vi "RT_DETR_OpenVINO.vi"() -> ()   [LabVIEW 2018]
doc: "RT_DETR_OpenVINO: This example is an object detection example of the RT-DETR algorithm, which can perform object detection on real-time images captured by cameras."
uses:
  vi.lib/VIRobotics/opencv_yiku/Cap/Cap.lvclass
  vi.lib/VIRobotics/ModelZoo/Object_Detection/RT_DETR_OpenVINO/RT_DETR_OpenVINO.lvclass
  vi.lib/VIRobotics/opencv_yiku/Mat/Mat_8U/Mat_8U.lvclass
panel:
  in  "config":T1={"confThreshold"=0.3, "nms_threshold"=0.5, "fontScale"=0.5}
  in  "device_name":string(combo)="CPU"
  in  "model_file":path=path "C:/ProgramData/VIRobotics/ModelZoo/Object_Detection/RT_DETR/onnx_model/rtdetr_r50vd_m_6x_coco.onnx"
  in  "class_names_file":path=path "C:/ProgramData/VIRobotics/ModelZoo/Object_Detection/coco.names"
  out "每帧耗时(s)":dbl
  in  "stop":bool
  out "picture":picture
  # "Overview: Demonstrates how to use OpenVINO to load the the ONNX model of pp-rtdetr for real-time object detection.\nRequirements: Windows.\nMake sure your computer has a camera。\nInstructions: \nIf you want to load the model, follow the following steps:\n1.Select the device_name to use. \n2.Specify the model_file and class_names_file.(Because the model is too large, it is not loaded by default.)\n3.Run the VI."
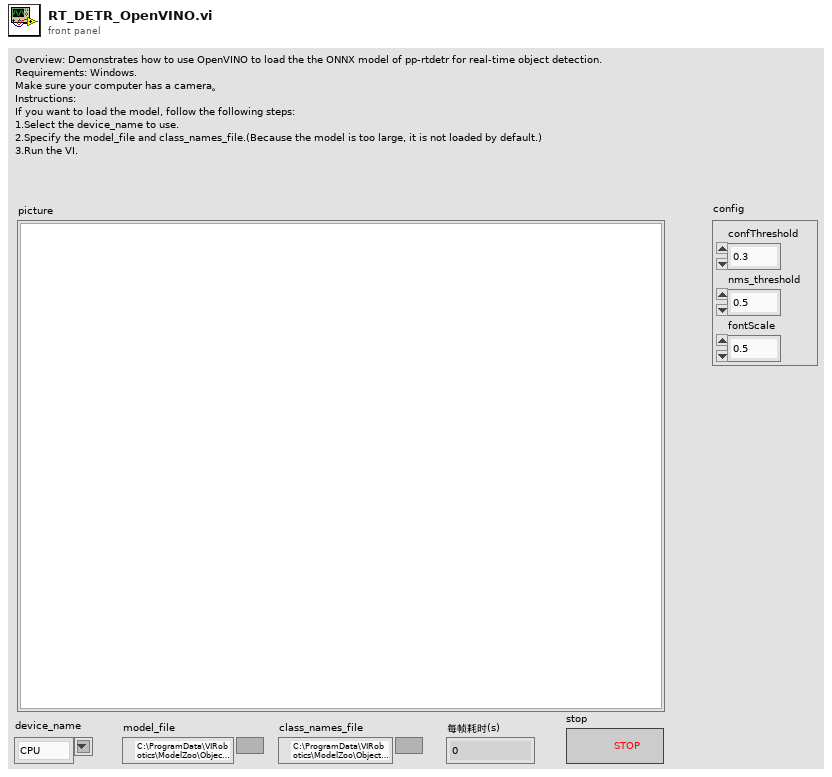
[diagram p1: front panel]
types:
  T1 = cluster{"confThreshold":sgl, "nms_threshold":sgl, "fontScale":dbl}
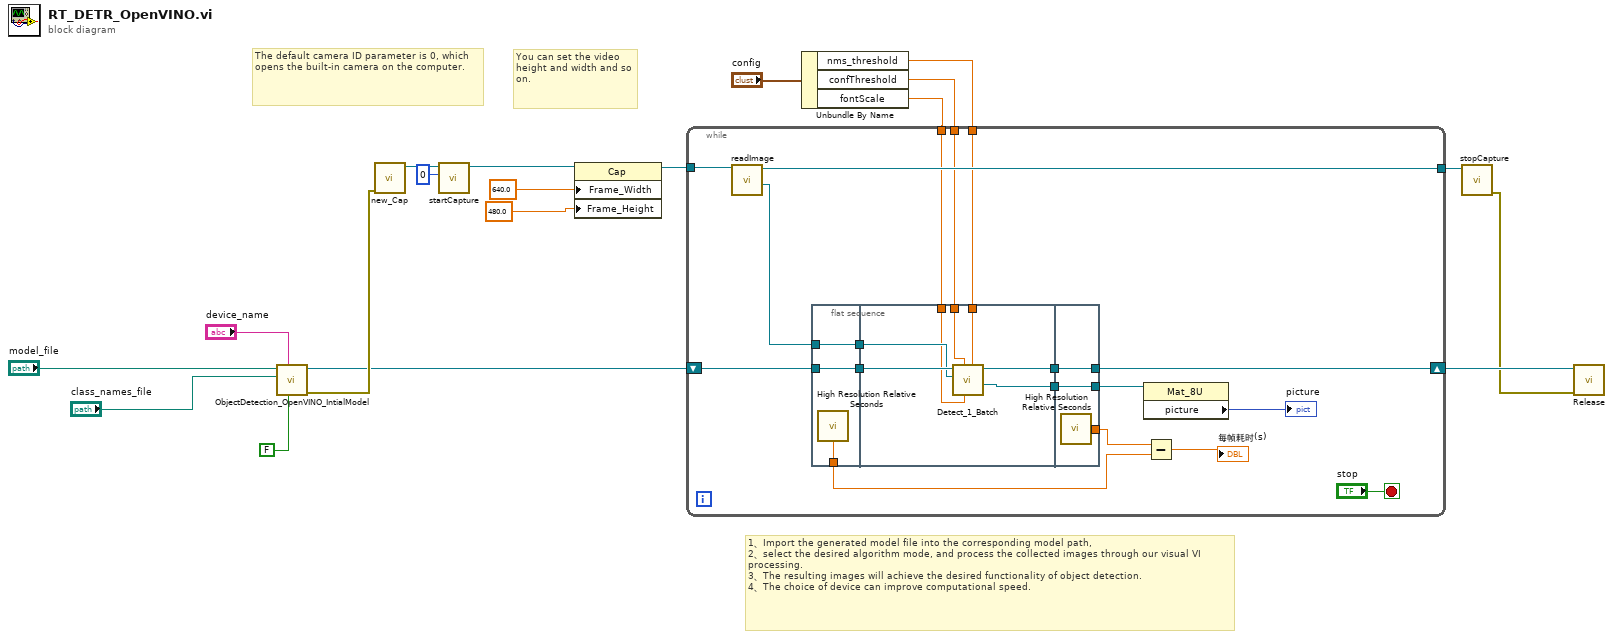
[diagram p0: block diagram]
diagram:
  # "1、Import the generated model file into the corresponding model path, \n2、select the desired algorithm mode, and process the collected images through our visual VI processing. \n3、The resulting images will achieve the desired functionality of object detection. \n4、The choice of device can improve computational speed."
  # "You can set the video height and width and so on."
  # "The default camera ID parameter is 0, which opens the built-in camera on the computer."
  n1 = call-poly "ObjectDetection_OpenVINO_IntialModel.vi"("use letterbox"=FALSE, "device_name"="device_name", "class_names_path"="class_names_file", "onnx_file"="model_file") -> ("error out"=w11:errorcluster, "detr_ov out"=w7:refnum<class "RT_DETR_OpenVINO.lvclass">)  [unwired: 6 in]
  n2 = call "new_Cap.vi"("error in (no error)"=w11) -> ("Cap out"=w18:refnum<class "Cap.lvclass">)  [unwired: 9 in, 1 out]
  n3 = call "startCapture.vi"("cameraID"=0, "Cap in"=w18) -> ("Cap out"=w17:refnum<class "Cap.lvclass">)  [unwired: 8 in, 1 out]
  n4 = property class="Cap"(reference=w17, "Frame_Width"=640.0, "Frame_Height"=480.0) -> (reference out=w14:refnum<class "Cap.lvclass">)  [unwired: 1 in, 1 out]
  n5 = Unbundle By Name("config") -> ("nms_threshold"=w3:sgl, "confThreshold"=w2:sgl, "fontScale"=w1:dbl)
  n6 = while {
    shift-right: [w33] -> w19
    shift-left: w7 -> [w37]
    tunnel: w14 -> [w25]
    tunnel: [w24] -> w13
    tunnel: w3 -> [w22]
    tunnel: w2 -> [w21]
    tunnel: w1 -> [w20]
    stop <- "stop" stop-if-true
    n7 = call "readImage.vi"("Cap in"=w25) -> ("Mat out"=w23:refnum<class "Mat_8U.lvclass">, "Cap out"=w24:refnum<class "Cap.lvclass">)  [unwired: 8 in, 1 out]
    n8 = flat-sequence {
      tunnel: w23 -> [w39]
      tunnel: w37 -> [w40]
      tunnel: [w40] -> w32
      tunnel: [w39] -> w31
      tunnel: [w38] -> w27
      tunnel: w32 -> [w47]
      tunnel: w31 -> [w44]
      tunnel: [w46] -> w30
      tunnel: [w45] -> w29
      tunnel: w22 -> [w43]
      tunnel: w21 -> [w42]
      tunnel: w20 -> [w41]
      tunnel: [w49] -> w33
      tunnel: [w50] -> w36
      tunnel: w30 -> [w50]
      tunnel: w29 -> [w49]
      tunnel: [w48] -> w28
      frame #0 {
        n9 = call <vilib>:"High Resolution Relative Seconds.vi"() -> ("relative seconds"=w38:dbl)
      }
      frame #1 {
        n10 = call-dynamic "Detect_1_Batch.vi"("nms_threshold"=w43, "fontScale"=w41, "confThreshold"=w42, "image"=w44, "RT_DETR_OpenVINO in"=w47) -> ("img out"=w46:refnum<class "Mat_8U.lvclass">, "RT_DETR_OpenVINO out"=w45:refnum<class "RT_DETR_OpenVINO.lvclass">)  [unwired: 3 in, 2 out]
      }
      frame #2 {
        n11 = call <vilib>:"High Resolution Relative Seconds.vi"() -> ("relative seconds"=w48:dbl)
      }
    }
    n12 = property class="Mat_8U"(reference=w36) -> ("picture"=→"picture":picture)  [unwired: 1 in, 2 out]
    n13 = Subtract(x=w28, y=w27) -> (x-y=→"每帧耗时(s)":dbl)
  }
  n14 = call "stopCapture.vi"("Cap in"=w13) -> ("error out"=w12:errorcluster)  [unwired: 10 in]
  n15 = call-dynamic "Release.vi"("error in (no error)"=w12, "RT_DETR_OpenVINO in"=w19) -> ()  [unwired: 8 in, 2 out]
